vi "create_day_folder.vi"(11 "Root folder":string="D:\\Michael Lohmann\\Messungen\\") -> (0 "Error Out":errorcluster, 3 "Day Folder":string)   [LabVIEW 2009]
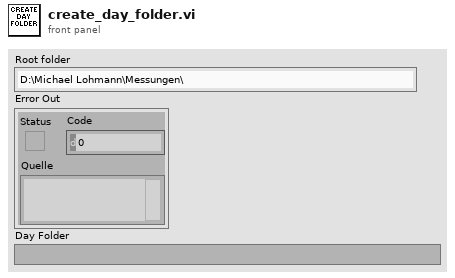
[diagram p1: front panel]
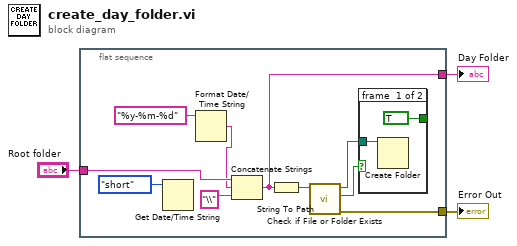
[diagram p0: block diagram]
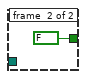
[diagram p2: hidden frame]
diagram:
  n1 = flat-sequence {
    tunnel: [w13] -> w3
    tunnel: [w12] -> w2
    tunnel: "Root folder" -> [w8]
    frame #0 {
      n2 = Get Date/Time String(date format (0)=enum16{"short", "long", "abbreviated"}."short" ("Datumsformat (0)")) -> ()  [unwired: 2 in, 2 out]
      n3 = Format Date/Time String(time format string (%c)="%y-%m-%d" ("Zeitformatierungs-String (%c)")) -> (date/time string=w4:string)  [unwired: 2 in]
      n4 = Concatenate Strings(w8, w4, "\\" ("String")) -> (w13:string)
      n5 = String To Path(string=w13) -> (path=w11:path)
      n6 = call <vilib>:"Check if File or Folder Exists.vi"("path"=w11) -> ("error out"=w12:errorcluster, "file or folder exists?"=w10:bool, "dup path"=w9:path)  [unwired: 8 in]
      n7 = case shown="False" w10 {
        tunnel: w9 -> [w15 _]
        tunnel: [TRUE FALSE] -> _
        frame #0 {
          n8 = Create Folder(path (use dialog)=w15) -> ()  [unwired: 2 in, 3 out]
        }
        frame #1 {
        }
      }
    }
  }
  "Day Folder" <- w3
  "Error Out" <- w2
